vi "Apply Leverage Force.vi"(10 "force":dbl, 11 "Box in":refnum<class "Box.lvclass">) -> (3 "Box out":refnum<class "Box.lvclass">)   [LabVIEW 2023, in "Box.lvclass"]
uses:
  Box.lvclass
  Box State.ctl
  Box.lvclass/Box.ctl
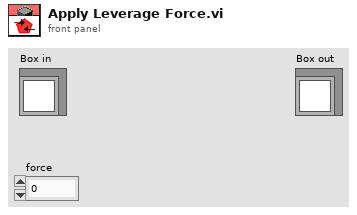
[diagram p1: front panel]
types:
  T1 = typedef "Box.lvclass/Box State.ctl" = enum16{"Closed", "Open"}
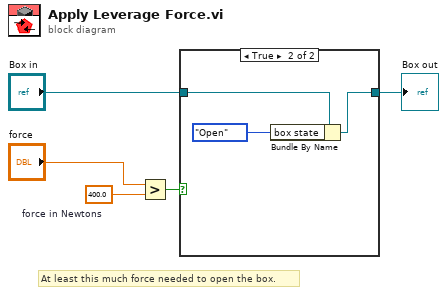
[diagram p0: block diagram]
diagram:
  w4 = 400.0  # force in Newtons
  # "At least this much force needed to open the box."
  n1 = Greater?(x="force", y=w4) -> (0:w3:bool)
  n2 = case shown="True" w3 {
    tunnel: "Box in" -> [w6 w9]
    tunnel: [w6 w7] -> w1
    frame False {
    }
    frame True {
      n3 = Bundle By Name(cluster=w9, "box state"=Box_State."Open") -> (w7:refnum<class "Box.lvclass">)
    }
  }
  "Box out" <- w1
